vi "Send VISA Command.vi"(8 "error in (no error)":errorcluster, 10 "Command":string, 11 "336XX in":refnum<class "336XX.lvclass">) -> (0 "error out":errorcluster, 3 "336XX out":refnum<class "336XX.lvclass">)   [LabVIEW 2019, in "336XX.lvlib" / "336XX.lvclass"]
uses:
  Library/336XX.lvclass
  Library/336XX.lvclass/336XX.ctl
  <instrlib>/Agilent 3352X Series/Agilent 3352X Series.lvlib
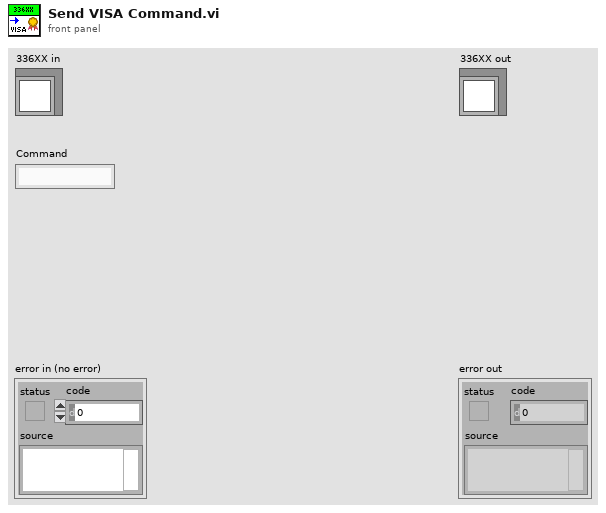
[diagram p1: front panel]
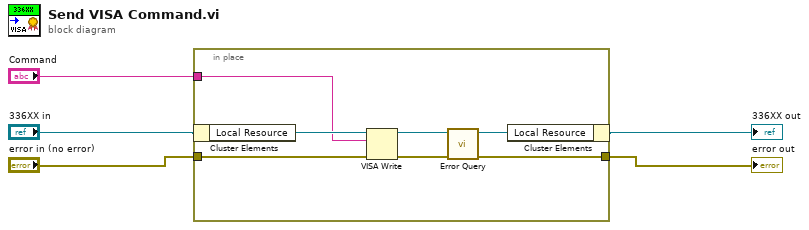
[diagram p0: block diagram]
diagram:
  n1 = in-place {
    in-place-border: "error in (no error)" -> [w8]
    in-place-border: [w7] -> w2
    in-place-border: "Command" -> [w6]
    n2 = in-place-cluster #1("336XX in") -> ("Local Resource"=w11:refnum<visa-resource-name>)
    n3 = VISA Write(VISA resource name=w11, write buffer=w6, error in (no error)=w8) -> (VISA resource name out=w10:refnum<visa-resource-name>, error out=w9:errorcluster)  [unwired: 1 out]
    n4 = call <instrlib>:"Error Query.vi"("error in (no error)"=w9, "VISA resource name"=w10) -> ("error out"=w7:errorcluster, "VISA resource name out"=w12:refnum<visa-resource-name>)  [unwired: 8 out]
    n5 = in-place-cluster #1("Local Resource"=w12) -> (→"336XX out":refnum<class "336XX.lvclass">)
  }
  "error out" <- w2
